vi "main_agv_old.vi"() -> ()   [LabVIEW 2018]
uses:
  Ctrl/SoutWork.ctl
  Ctrl/gps-232.ctl
  Ctrl/gps-databuf.ctl
  Ctrl/obstacle_info.ctl
  Ctrl/waypoint_buf.ctl
  Subvi/global_setting.vi
  <vilib>/imath/engines/lvmath2/RunTimeEngine/Managers/WorkSpace/UID Generator.vi
  <vilib>/imath/engines/lvmath2/RunTimeEngine/RunTimeType/NIMS_RunTimeType_From StrictType (excl LVString).vi
  <instcachedir>/0/NIMS_RunTimeType_From StrictType (excl LVString)_E7E34A65C99947108168652BAD14964D.lvgen/NIMS_RunTimeType_From StrictType (excl LVString)_E7E34A65C99947108168652BAD14964D_000.vi
  <vilib>/imath/engines/lvmath2/RunTimeEngine/LocalVariableDefStatement/MC_LocalVariableDefStatement_Display.vi
  <vilib>/imath/engines/lvmath2/RunTimeEngine/Managers/SymbolTable/Clear UID.vi
  <vilib>/imath/engines/lvmath2/RunTimeEngine/NodeEndStatement/NIMS_NodeEndStatement_Output.vi
  <instcachedir>/0/NIMS_NodeEndStatement_Output_53EC0D466D134D7ABD903AC30B43404B.lvgen/NIMS_NodeEndStatement_Output_53EC0D466D134D7ABD903AC30B43404B_001.vi
  <vilib>/imath/engines/lvmath2/RunTimeEngine/ErrorHandling/NIMS_Finalize Error.vi
  <vilib>/imath/engines/lvmath2/RunTimeEngine/Managers/SymbolTable/NIMS_WorkSpace.lvlib
panel:
  in  "System status":string
  in  "tab":T1(tab)
  in  "starttest":bool
  out "System Feedback":T2={"system state"="normal", "Control Mode"=0, "Battery Voltage (V)"=27.3, "error code High"=0, "error code Low"=0}
  out "AGV_EStop":bool
  out "LiDAR":cluster{sgl[], sgl[]}[](graph)
  out "LiDAR img":T3(plugin-control)
  out "GPS XY Graph":cluster{"X1":dbl, "Y1":dbl}[](graph)
  out "Path":cluster{"pathF4.23":ext[], "pathF4.23":ext[]}[](graph)
  out "Manual":bool
  out "ChoosePath":bool
  out "PathFlag":bool
  out "Obstacle Stop":bool
  out "System Start/Stop":bool
  out "Remote_Stop":bool
  out "Motion Feedback":T4={"Linear Velocity (m/s)"=-0.982, "Angular Velocity (rad/s)"=-0.008} {"Linear Velocity (m/s)" format="%.2f"; "Angular Velocity (rad/s)" format="%.2f"}
  out "Vehicle Motion State":T5
  out "current index":dbl=1036.0 format="%#.1f"
  out "linear velocity":dbl=0.19999999999999996 format="%.2f"
  out "angular velocity":dbl=0.2222269923246912 format="%.2f"
  out "Rotational Vel (rad/s)":dbl min=0.0 max=1.0 step=0.001
  out "Translational Vel (m/s)":dbl min=-1.0 max=1.0 step=0.1
  out "heading=0 alarm":bool
  in  "obstacle limit range":T6={"RL front-x"=1.7, "RL central-x"=1.7, "front-y"=2.0} {"front-y" format="%.1f"}
  out "Image":T3(plugin-control)
  in  "TIM571 IP":string="192.168.0.2"
  in  "TIM571 Mounting Offset":T7={"X_offset[m]"=0.0, "Y_offset[m]"=0.68, "Z_offset[m]"=0.0, "X_Rotation[Deg]"=0.0, "Y_Rotation[Deg]"=180.0, "Z_Rotation[Deg]"=0.0} {"Z_Rotation[Deg]" format="%#.2f"; "Y_Rotation[Deg]" format="%#.2f"; "X_Rotation[Deg]" format="%#.2f"; "Z_offset[m]" format="%#.2f"; "Y_offset[m]" format="%#.2f"; "X_offset[m]" format="%#.2f"}
  in  "vlp-16 range setting":T8={"x range"=20.0, "y range Max"=10.0, "y range Min"=-10.0, "z range"=1.0}
  in  "VLP16 Mounting Offset":T7 {"Z_Rotation[Deg]" format="%#.2f"; "Y_Rotation[Deg]" format="%#.2f"; "X_Rotation[Deg]" format="%#.2f"; "Z_offset[m]" format="%#.2f"; "Y_offset[m]" format="%#.2f"; "X_offset[m]" format="%#.2f"}
  out "LiDAR U8":u8[](array[numeric])
  out "232 buf n":u32(graph)
  out "Heading":dbl=98.684623718
  in  "baud rate gps":u32=115200
  in  "vehicle status":T9
  in  "AGV_Port":refnum<visa-resource-name>="COM5"
  out "Robot Status":T9={"X (m)"=153.55383758084335, "Y (m)"=122.1653462474019, "Z (m)"=9.9059, "Roll (degree)"=-0.425709275, "Pitch (degree)"=-0.898393069, "Heading (degree)"=-8.684623717999997, "Linear velocity (m/s)"=-0.982, "Angular velocity (rad/s)"=-0.008} {"X (m)" format="%.2f"; "Y (m)" format="%#.2f"; "Z (m)" format="%#.2f"; "Roll (degree)" format="%_2g"; "Pitch (degree)" format="%.2f"; "Heading (degree)" format="%.2f"; "Linear velocity (m/s)" format="%.2f"; "Angular velocity (rad/s)" format="%.2f"}
  in  "Remote PC IP":string="223.171.61.153"
  out "Resources":string[][](table)
  out "waypoint graph":T10(graph)
  in  "pathF4.23":ext[][](array[numeric])=array2x4344[8688 elements]
  in  "P2F":ext[][](array[numeric])=array2x2176[4352 elements]
  in  "P1F":ext[][](array[numeric])=array2x2168[4336 elements]
  out "index Y":ext
  out "index X":ext
  out "GNSS Error":errorcluster
  out "IndexPath":ext[][](array[numeric])
  out "Frames/Sec 3":dbl=50.026287540850646 format="%#_2g"
  out "System Feedback code":u8[](array[numeric])=[0, 0, 1, 17, 0, 0]
  out "GPS Data":T11={"Latitude"={"Valid?"=TRUE, "Latitude (Deg)"=37.37123095061}, "Longitude"={"Valid?"=TRUE, "Longitude (Deg)"=126.72256864175}, "Height"={"Valid?"=TRUE, "Height (m)"=9.9059}, "Undulation"={"Valid?"=TRUE, "Undulation(m)"=22.3}, "North Vel"={"Valid?"=TRUE, "North Vel (m/s)"=-0.0013}, "East Vel"={"Valid?"=TRUE, "East Vel (m/s)"=-0.002}, "Up Vel"={"Valid?"=TRUE, "Up Vel (m/s)"=0.0004}, "Roll"={"Valid?"=TRUE, "Roll (degrees)"=-0.425709275}, "Pitch"={"Valid?"=TRUE, "Pitch (degrees)"=-0.898393069}, "Azimuth"={"Valid?"=TRUE, "Azimuth (degrees)"=98.594488749}, "Lat deviation"={"Valid?"=TRUE, "Lat deviation (m)"=0.4755}, "Long deviation"={"Valid?"=TRUE, "Long deviation (m)"=0.4754}, "Height deviation"={"Valid?"=TRUE, "Height deviation (m)"=0.9034}, "North vel deviation"={"Valid?"=TRUE, "North vel deviation (m/s)"=0.0181}, "East vel deviation"={"Valid?"=TRUE, "East vel deviation (m/s)"=0.018}, "Up vel deviation"={"Valid?"=TRUE, "Up vel deviation (m/s)"=0.0196}, "Roll deviation"={"Valid?"=TRUE, "Roll deviation (degrees)"=0.0309}, "Pitch deviation"={"Valid?"=TRUE, "Pitch deviation (degrees)"=0.0311}, "Azimuth deviation"={"Valid?"=TRUE, "Azimuth deviation (degrees)"=0.1368}, "Ext sol status"={"Valid?"=TRUE, "Ext sol status"=0.0}}
  in  "stop":bool
  # "GNSS"
  # "Mando Patrol robot"
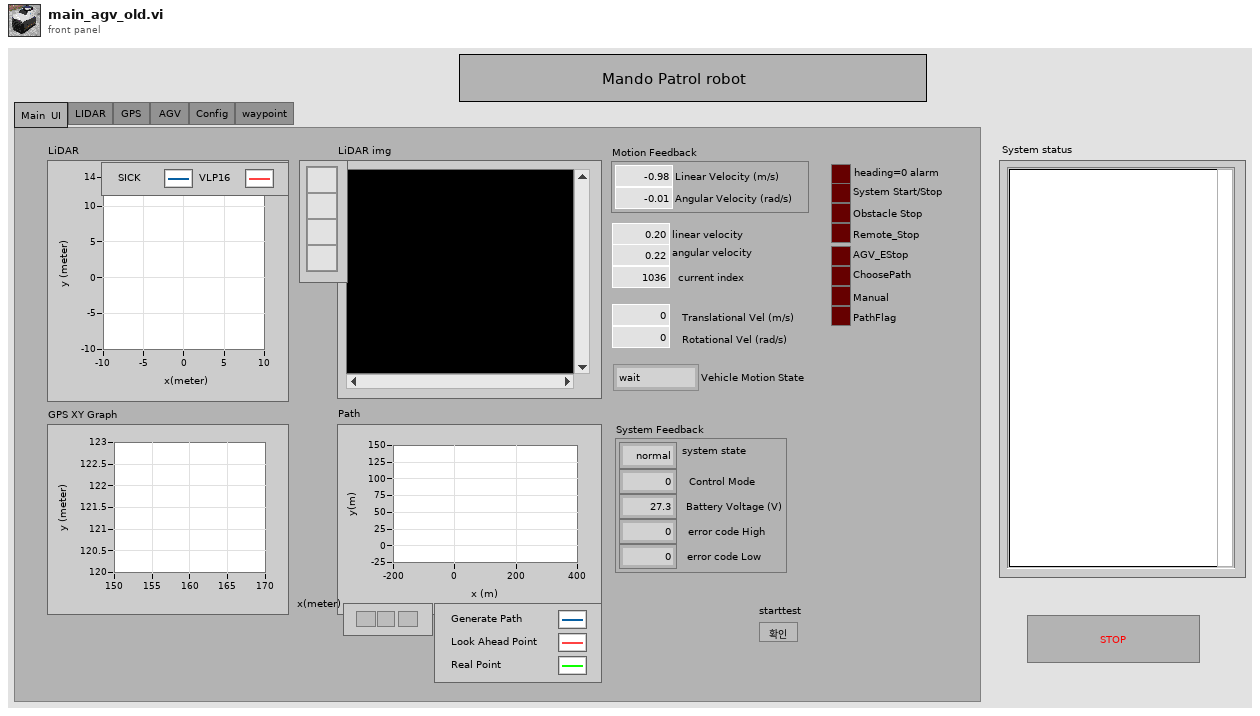
[diagram p1: front panel]
types:
  T1 = enum32{"Main  UI", "LIDAR", "GPS ", "AGV ", "Config", "waypoint"}
  T2 = cluster{"system state":string, "Control Mode":u8, "Battery Voltage (V)":dbl, "error code High":u8, "error code Low":u8}
  T3 = typedef "IMAQ Image.ctl" = refnum<image>
  T4 = cluster{"Linear Velocity (m/s)":dbl, "Angular Velocity (rad/s)":dbl}
  T5 = typedef "SoutWork.ctl" = enum16{"wait", "Move", "ObstacleStop", "EStop", "Goal"}
  T6 = cluster{"RL front-x":dbl, "RL central-x":dbl, "front-y":dbl}
  T7 = cluster{"X_offset[m]":sgl, "Y_offset[m]":sgl, "Z_offset[m]":sgl, "X_Rotation[Deg]":sgl, "Y_Rotation[Deg]":sgl, "Z_Rotation[Deg]":sgl}
  T8 = cluster{"x range":dbl, "y range Max":dbl, "y range Min":dbl, "z range":dbl}
  T9 = cluster{"X (m)":dbl, "Y (m)":dbl, "Z (m)":dbl, "Roll (degree)":dbl, "Pitch (degree)":dbl, "Heading (degree)":dbl, "Linear velocity (m/s)":dbl, "Angular velocity (rad/s)":dbl}
  T10 = cluster{"waypoint out":cluster{"x":dbl, "y":dbl}[]}[]
  T11 = cluster{"Latitude":cluster{"Valid?":bool, "Latitude (Deg)":dbl}, "Longitude":cluster{"Valid?":bool, "Longitude (Deg)":dbl}, "Height":cluster{"Valid?":bool, "Height (m)":dbl}, "Undulation":cluster{"Valid?":bool, "Undulation(m)":dbl}, "North Vel":cluster{"Valid?":bool, "North Vel (m/s)":dbl}, "East Vel":cluster{"Valid?":bool, "East Vel (m/s)":dbl}, "Up Vel":cluster{"Valid?":bool, "Up Vel (m/s)":dbl}, "Roll":cluster{"Valid?":bool, "Roll (degrees)":dbl}, "Pitch":cluster{"Valid?":bool, "Pitch (degrees)":dbl}, "Azimuth":cluster{"Valid?":bool, "Azimuth (degrees)":dbl}, "Lat deviation":cluster{"Valid?":bool, "Lat deviation (m)":dbl}, "Long deviation":cluster{"Valid?":bool, "Long deviation (m)":dbl}, "Height deviation":cluster{"Valid?":bool, "Height deviation (m)":dbl}, "North vel deviation":cluster{"Valid?":bool, "North vel deviation (m/s)":dbl}, "East vel deviation":cluster{"Valid?":bool, "East vel deviation (m/s)":dbl}, "Up vel deviation":cluster{"Valid?":bool, "Up vel deviation (m/s)":dbl}, "Roll deviation":cluster{"Valid?":bool, "Roll deviation (degrees)":dbl}, "Pitch deviation":cluster{"Valid?":bool, "Pitch deviation (degrees)":dbl}, "Azimuth deviation":cluster{"Valid?":bool, "Azimuth deviation (degrees)":dbl}, "Ext sol status":cluster{"Valid?":bool, "Ext sol status":dbl}}
  T12 = typedef "gps-232.ctl" = enum16{"ini", "timing set", "read", "write", "close"}
  T13 = enum16{"write mounting offset", "write range setting", "read"}
  T14 = typedef "obstacle_info.ctl" = enum16{"init", "read", "obstacle status in", "write limit"}
  T15 = typedef "operation.ctl" = enum16{"init", "move", "start pt", "end pt", "start heading adjust", "move heading adjust"}
  T16 = cluster{"VLP16":cluster{"Range setting":cluster{"x range":dbl, "y range Max":dbl, "y range Min":dbl, "z range":dbl}, "Mounting Offset":cluster{"X_offset[m]":sgl, "Y_offset[m]":sgl, "Z_offset[m]":sgl, "X_Rotation[Deg]":sgl, "Y_Rotation[Deg]":sgl, "Z_Rotation[Deg]":sgl}}, "TIM571":cluster{"TIM571 IP":string, "TIM571 Mounting Offset":cluster{"X_offset[m]":sgl, "Y_offset[m]":sgl, "Z_offset[m]":sgl, "X_Rotation[Deg]":sgl, "Y_Rotation[Deg]":sgl, "Z_Rotation[Deg]":sgl}}, "Devices":string[][], "Scout":cluster{"scout port":refnum<visa-resource-name>, "limit_linear-v":dbl, "limit_angular-v":dbl}, "PwrPak7":cluster{"PwrPak7 port":refnum<visa-resource-name>}, "PID":cluster{"PID gains":cluster{"proportional gain (Kc)":dbl, "integral time (Ti, min)":dbl, "derivative time (Td, min)":dbl}, "PID limits":cluster{"output high":dbl, "output low":dbl}, "dt pid":i64}, "Waypoint":cluster{"lookahead pts n":dbl, "lookahead length":dbl}, "obstacle limit range":cluster{"RL front-x":dbl, "RL central-x":dbl, "front-y":dbl}, "System state":cluster{"angle adjust limit":dbl, "State":T15}}
  T17 = cluster{"TIM571 IP":string, "TIM571 Mounting Offset":cluster{"X_offset[m]":sgl, "Y_offset[m]":sgl, "Z_offset[m]":sgl, "X_Rotation[Deg]":sgl, "Y_Rotation[Deg]":sgl, "Z_Rotation[Deg]":sgl}}
  T18 = cluster{"Translational Vel (m/s)":dbl, "Rotational Vel (rad/s)":dbl}
  T19 = cluster{"linear velocity":dbl, "angular velocity":dbl}
  T20 = typedef "gps-databuf.ctl" = enum16{"read", "write"}
  T21 = typedef "waypoint_buf.ctl" = enum16{"clear", "write", "read"}
  T22 = cluster{"rawdata":string, "GPS Data":cluster{"Latitude":cluster{"Valid?":bool, "Latitude (Deg)":dbl}, "Longitude":cluster{"Valid?":bool, "Longitude (Deg)":dbl}, "Height":cluster{"Valid?":bool, "Height (m)":dbl}, "Undulation":cluster{"Valid?":bool, "Undulation(m)":dbl}, "North Vel":cluster{"Valid?":bool, "North Vel (m/s)":dbl}, "East Vel":cluster{"Valid?":bool, "East Vel (m/s)":dbl}, "Up Vel":cluster{"Valid?":bool, "Up Vel (m/s)":dbl}, "Roll":cluster{"Valid?":bool, "Roll (degrees)":dbl}, "Pitch":cluster{"Valid?":bool, "Pitch (degrees)":dbl}, "Azimuth":cluster{"Valid?":bool, "Azimuth (degrees)":dbl}, "Lat deviation":cluster{"Valid?":bool, "Lat deviation (m)":dbl}, "Long deviation":cluster{"Valid?":bool, "Long deviation (m)":dbl}, "Height deviation":cluster{"Valid?":bool, "Height deviation (m)":dbl}, "North vel deviation":cluster{"Valid?":bool, "North vel deviation (m/s)":dbl}, "East vel deviation":cluster{"Valid?":bool, "East vel deviation (m/s)":dbl}, "Up vel deviation":cluster{"Valid?":bool, "Up vel deviation (m/s)":dbl}, "Roll deviation":cluster{"Valid?":bool, "Roll deviation (degrees)":dbl}, "Pitch deviation":cluster{"Valid?":bool, "Pitch deviation (degrees)":dbl}, "Azimuth deviation":cluster{"Valid?":bool, "Azimuth deviation (degrees)":dbl}, "Ext sol status":cluster{"Valid?":bool, "Ext sol status":dbl}}, "Heading":dbl, "utm-1":cluster{"XN":dbl, "YE":dbl}}
  T23 = cluster{"Latitude (Deg)":dbl, "Longitude (Deg)":dbl}
  T24 = cluster{"waypoint out":cluster{"x":dbl, "y":dbl}[]}
  T25 = cluster{"waypoint out":cluster{"Y(E)":dbl, "X(N)":dbl}[]}[]
  T26 = cluster{u8, "index X":ext, "index Y":ext, "System Start/Stop":bool}
  T27 = cluster{"Real Matrix Element":dbl, "Real Matrix Element":dbl}
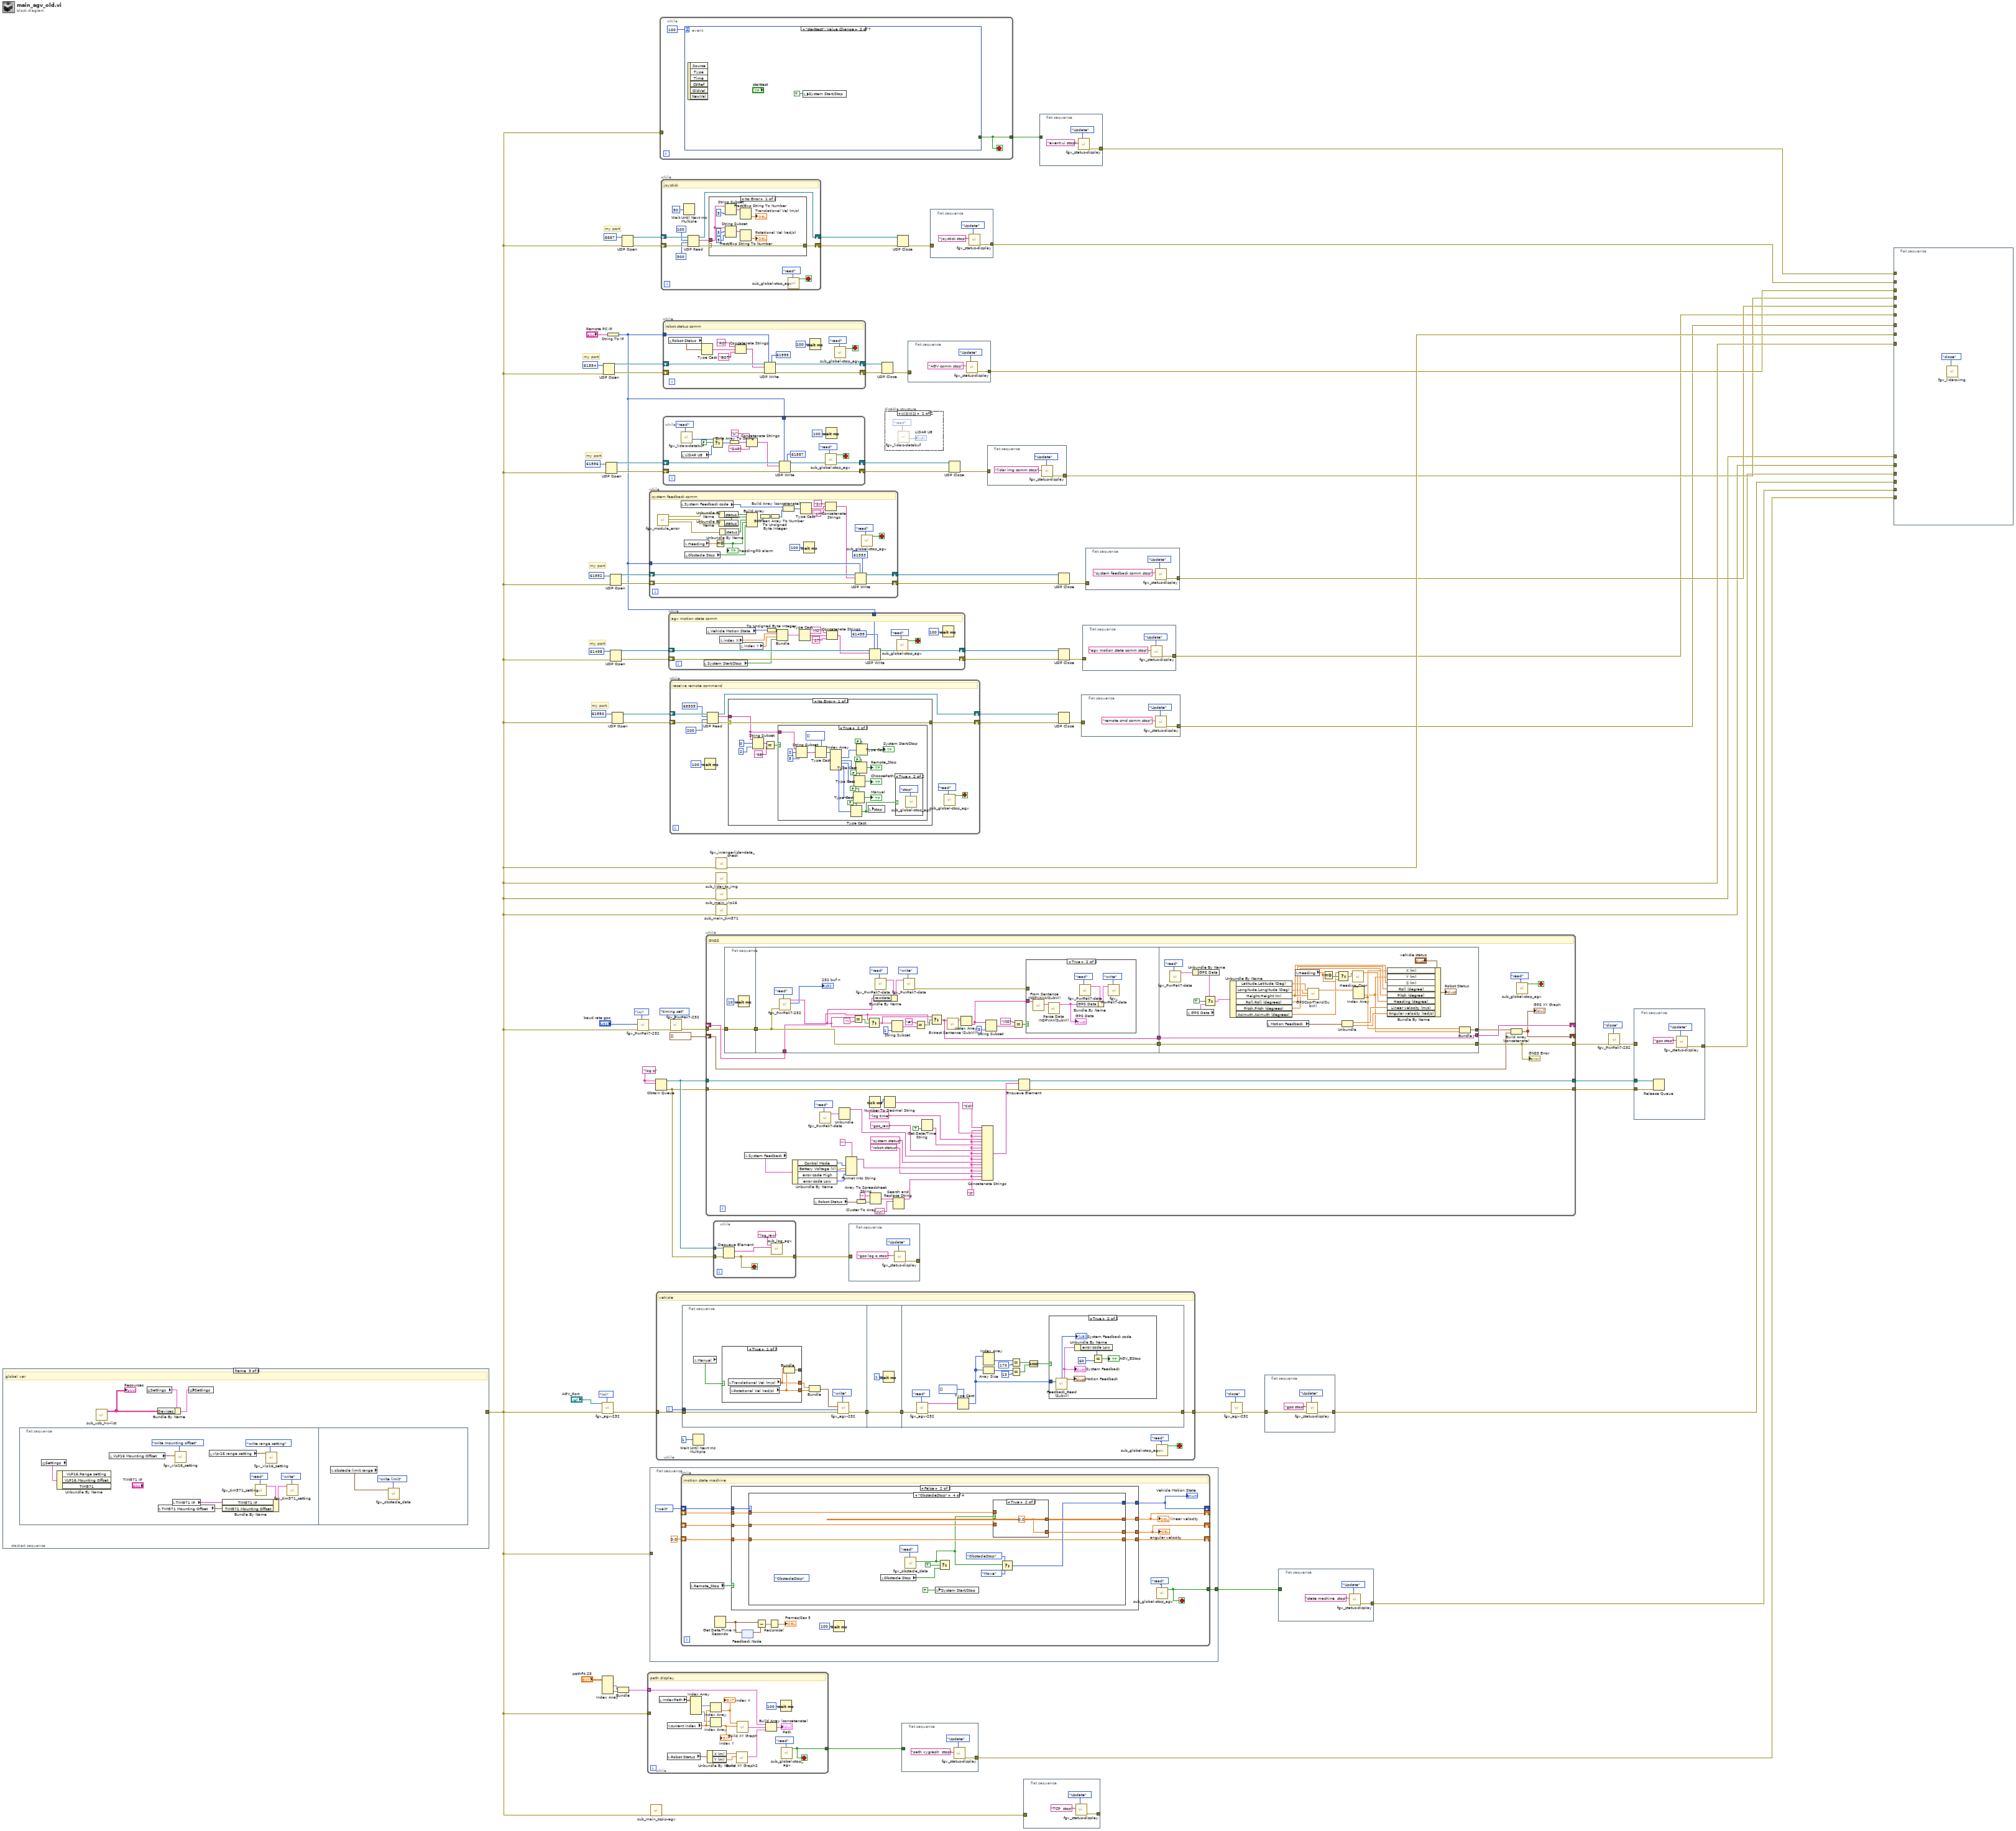
[diagram p0: block diagram]
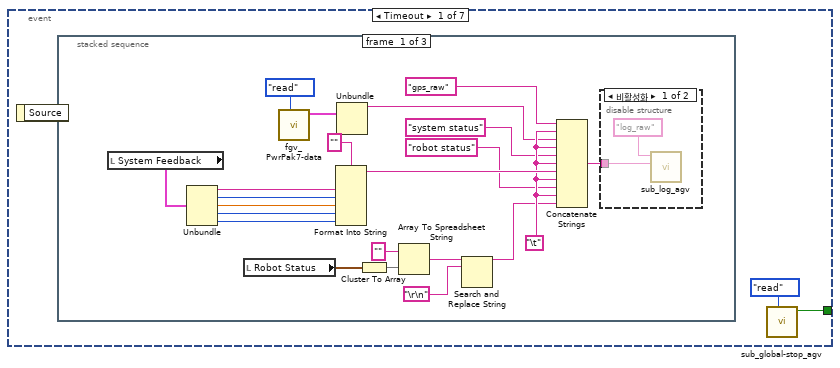
[diagram p3: hidden frame]
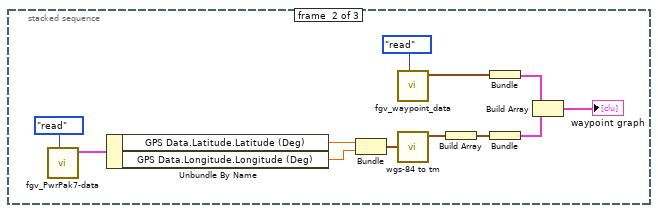
[diagram p5: hidden frame]
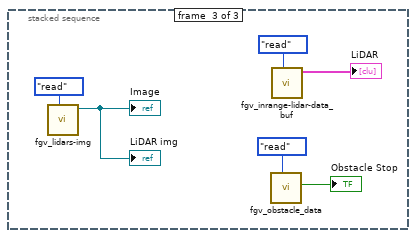
[diagram p6: hidden frame]
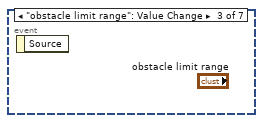
[diagram p7: hidden frame]
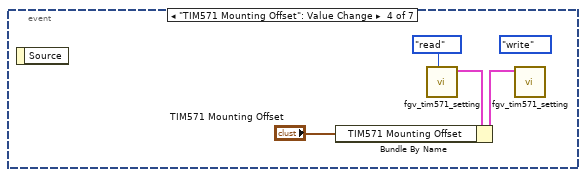
[diagram p8: hidden frame]
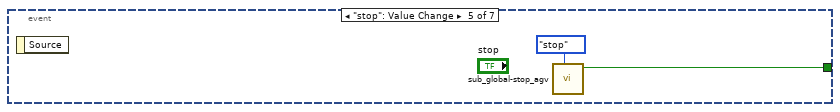
[diagram p9: hidden frame]
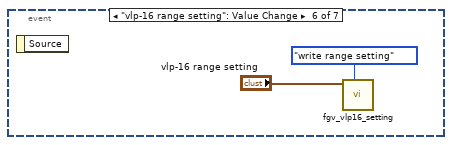
[diagram p10: hidden frame]
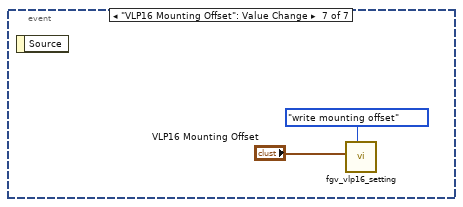
[diagram p11: hidden frame]
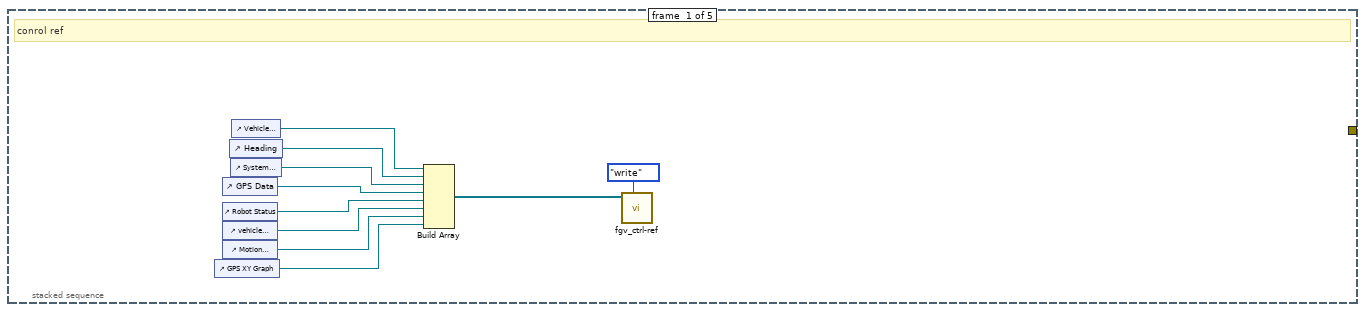
[diagram p12: hidden frame]
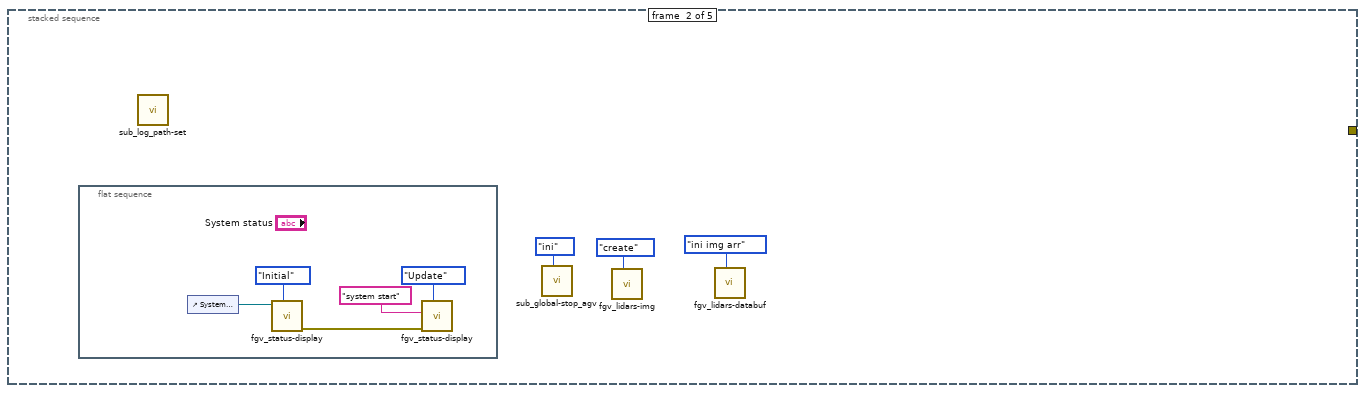
[diagram p13: hidden frame]
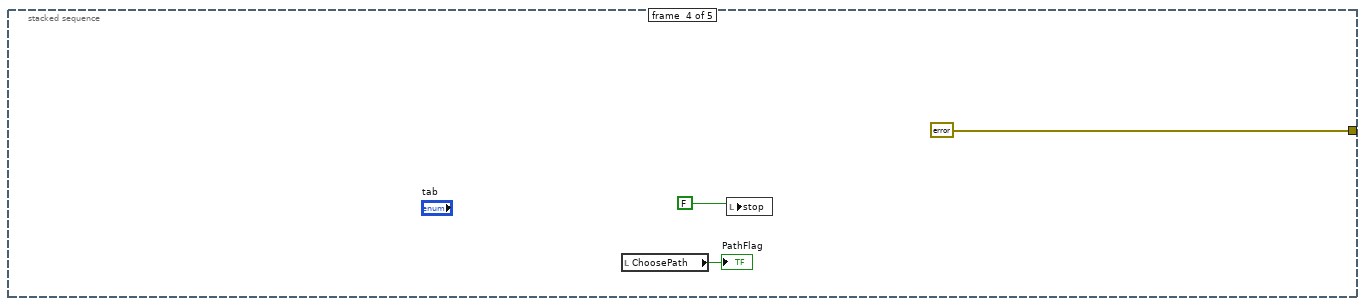
[diagram p14: hidden frame]
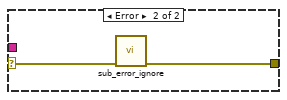
[diagram p16: hidden frame]
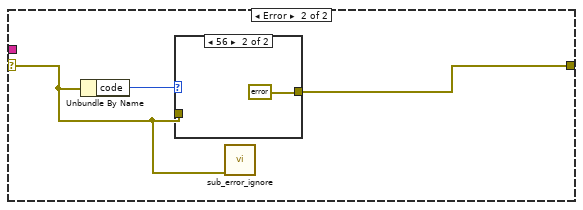
[diagram p19: hidden frame]
diagram:
  w4 = "log q" ("이름(이름없음)")
  # "my port"
  # "my port"
  # "my port"
  # "my port"
  # "my port"
  # "my port"
  n1 = stacked-sequence {
    tunnel: [_ _ _ errorcluster {"status"=FALSE, "code"=0, "source"=""} ("error in (no error)") _] -> w3
    frame #0 {
      # "conrol ref"
      n2 = control-ref of="GPS XY Graph"() -> (w91:refnum<vi>)
      n3 = control-ref of="GPS Data"() -> (w89:refnum<vi>)
      n4 = control-ref of="Robot Status"() -> (w88:refnum<vi>)
      n5 = control-ref of="vehicle status"() -> (w87:refnum<vi>)
      n6 = control-ref of="Motion Feedback"() -> (w90:refnum<vi>)
      n7 = control-ref of="Heading"() -> (w93:refnum<vi>)
      n8 = control-ref of="System status"() -> (w92:refnum<vi>)
      n9 = control-ref of="Vehicle Motion State"() -> (w84:refnum<vi>)
      n10 = Build Array(w84, w93, w92, w89, w88, w87, w90, w91) -> (w86:refnum<vi>[])
      n11 = call "fgv_ctrl-ref.vi"("cmd"=enum16{"write", "read"}."write", "ctrl in"=w86) -> ()  [unwired: 9 in, 1 out]
    }
    frame #1 {
      n12 = flat-sequence {
        frame #0 {
          n13 = control-ref of="System status"() -> (w101:refnum<vi>)
          n14 = call "fgv_status-display.vi"("Mode"=enum16{"Initial", "Update", "Clear"}."Initial", "System Log"=w101) -> ("error out"=w100:errorcluster)  [unwired: 9 in]
          n15 = call "fgv_status-display.vi"("Mode"=enum16{"Initial", "Update", "Clear"}."Update", "error in"=w100, "title"="system start" ("String in 1")) -> ()  [unwired: 8 in, 1 out]
        }
      }
      n16 = call "sub_log_path-set.vi"() -> ()  [unwired: 12 in]
      n17 = call "sub_global-stop_agv.vi"("cmd"=enum16{"ini", "read", "stop"}."ini") -> ()  [unwired: 10 in, 1 out]
      n18 = call "fgv_lidars-img.vi"("cmd"=enum16{"create", "read", "close"}."create") -> ()  [unwired: 10 in, 1 out]
      n19 = call "fgv_lidars-databuf.vi"("cmd"=enum16{"ini img arr", "write", "read"}."ini img arr") -> ()  [unwired: 9 in, 2 out]
    }
    frame #2 {
      # "global var"
      n20 = flat-sequence {
        frame #0 {
          n21 = global read "global_setting.vi" "Settings"() -> (w105:T16)
          n22 = Unbundle By Name(w105) -> ()  [unwired: 3 out]
          n23 = local read "VLP16 Mounting Offset"() -> (w114:T7)
          n24 = local read "TIM571 Mounting Offset"() -> (w109:T7)
          n25 = local read "TIM571 IP"() -> (w111:string)
          n26 = call "fgv_vlp16_setting.vi"("cmd"=T13."write mounting offset", "VLP16 Mounting Offset in"=w114) -> ()  [unwired: 7 in, 3 out]
          n27 = local read "vlp-16 range setting"() -> (w115:T8)
          n28 = call "fgv_tim571_setting.vi"("cmd"=enum16{"write", "read"}."read") -> ("tim571_setting-data_out"=w108:T17)  [unwired: 10 in]
          n29 = Bundle By Name(cluster=w108, "TIM571 IP"=w111, "TIM571 Mounting Offset"=w109) -> (w110:T17)
          n30 = call "fgv_vlp16_setting.vi"("cmd"=T13."write range setting", "vlp-16 range setting in"=w115) -> ()  [unwired: 7 in, 3 out]
          n31 = call "fgv_tim571_setting.vi"("cmd"=enum16{"write", "read"}."write", "tim571_setting-data_in"=w110) -> ()  [unwired: 9 in, 1 out]
        }
        frame #1 {
          n32 = local read "obstacle limit range"() -> (w116:T6)
          n33 = call "fgv_obstacle_data.vi"("cmd"=obstacle_info."write limit", "limit range"=w116) -> ()  [unwired: 7 in, 3 out]
        }
      }
      n34 = call "sub_usb_hw-list.vi"() -> ("Resources"=w104:string[][])  [unwired: 11 in]
      "Resources" <- w104
      n35 = global read "global_setting.vi" "Settings"() -> (w103:T16)
      n36 = Bundle By Name(cluster=w103, "Devices"=w104) -> (w102:T16)
      n37 = global write "global_setting.vi" "Settings"(w102) -> ()
    }
    frame #3 {
      n38 = local read "ChoosePath"() -> (→"PathFlag":bool)
      n39 = local write "stop"(FALSE ("stop")) -> ()
    }
    frame #4 {
    }
  }
  n40 = call "fgv_agv-232.vi"("cmd"=enum16{"ini", "write", "read", "close"}."ini", "error in"=w3, "COM Port"="AGV_Port") -> ("error out"=w78:errorcluster)  [unwired: 6 in, 2 out]
  n41 = Index Array(array="pathF4.23") -> (element #1=w53:ext[], element #2=w52:ext[])  [unwired: 4 in]
  n42 = UDP Open(8:w3, 11:u16 61554 ("port")) -> (port=w74:refnum<k16>, 0:w73:errorcluster)  [unwired: 3 in, 1 out]
  n43 = UDP Open(8:w3, 11:u16 61556 ("port")) -> (port=w80:refnum<k16>, 0:w79:errorcluster)  [unwired: 3 in, 1 out]
  n44 = String To IP(1:"Remote PC IP") -> (0:w49:u32)
  n45 = UDP Open(8:w3, 11:u16 61552 ("port")) -> (port=w68:refnum<k16>, 0:w67:errorcluster)  [unwired: 3 in, 1 out]
  n46 = UDP Open(8:w3, 11:u16 61498 ("port")) -> (port=w58:refnum<k16>, 0:w57:errorcluster)  [unwired: 3 in, 1 out]
  n47 = UDP Open(8:w3, 11:u16 61550 ("port")) -> (port=w63:refnum<k16>, 0:w62:errorcluster)  [unwired: 3 in, 1 out]
  n48 = Bundle("pathF4.23"=w53, "pathF4.23"=w52) -> (w54:cluster{"pathF4.23":ext[], "pathF4.23":ext[]})  [unwired: 1 in]
  n49 = UDP Open(8:w3, 11:u16 6667 ("port")) -> (port=w47:refnum<k16>, 0:w46:errorcluster)  [unwired: 3 in, 1 out]
  n50 = call "fgv_PwrPak7-232.vi"("cmd"=gps-232."ini", "error in"=w3, "baud rate"="baud rate gps") -> ("error out"=w16:errorcluster)  [unwired: 5 in, 3 out]
  n51 = while {
    tunnel: w54 -> [w135]
    tunnel: [w121] -> w31
    tunnel: w3 -> [_]
    stop <- w121 stop-if-true
    # "path display"
    n52 = local read "IndexPath"() -> (w127:ext[][])
    n53 = local read "Robot Status"() -> (w132:T9)
    n54 = local read "current index"() -> (w128:dbl)
    n55 = Index Array(array=w127) -> (element #1=w126:ext[], element #2=w125:ext[])  [unwired: 4 in]
    n56 = Unbundle By Name(w132) -> ("X (m)"=w131:dbl, "Y (m)"=w130:dbl)
    n57 = Index Array(array=w126, index=w128) -> (element=w124:ext)
    "index X" <- w124
    n58 = Index Array(array=w125, index=w128) -> (element=w123:ext)
    "index Y" <- w123
    n59 = call "Build XY Graph2"("Y Input"=w130, "X Input"=w131) -> ("XY Graph"=w129:cluster{"X":dbl[], "Y":dbl[]}[])  [unwired: 8 in, 1 out]
    n60 = call "Build XY Graph"("Y Input"=w123, "X Input"=w124) -> ("XY Graph"=w133:cluster{"X":dbl[], "Y":dbl[]}[])  [unwired: 8 in, 1 out]
    n61 = Build Array (concatenate)(w135, w133, w129) -> (→"Path":cluster{"pathF4.23":ext[], "pathF4.23":ext[]}[])
    n62 = Wait (ms)(milliseconds to wait=u32 100) -> ()  [unwired: 1 out]
    n63 = call "sub_global-stop_agv.vi"("cmd"=enum16{"ini", "read", "stop"}."read") -> ("stop status"=w121:bool)  [unwired: 10 in]
  }
  n64 = while {
    tunnel: w49 -> [w163]
    shift-right: [w160] -> w66
    shift-left: w68 -> [w162]
    shift-right: [w159] -> w65
    shift-left: w67 -> [w161]
    stop <- w140 stop-if-true
    # "system feedback comm"
    n65 = call "fgv_module_error.vi"() -> ("PwrPak7 error out"=w137:errorcluster, "tim571 error out"=w138:errorcluster, "vlp16 error out"=w139:errorcluster)  [unwired: 9 in]
    n66 = local read "System Feedback code"() -> (w153:u8[])
    n67 = local read "Heading"() -> (w145:dbl)
    n68 = local read "Obstacle Stop"() -> (w143:bool)
    n69 = Equal To 0?(x=w145) -> (x = 0?=w144:bool)
    "heading=0 alarm" <- w144
    n70 = Unbundle By Name(w139) -> ("status"=w157:bool)
    n71 = Unbundle By Name(w138) -> ("status"=w156:bool)
    n72 = Unbundle By Name(w137) -> ("status"=w146:bool)
    n73 = Build Array(w157, w156, w146, w144, w143) -> (w155:bool[])
    n74 = Boolean Array To Number(Boolean array=w155) -> (number=w154:u32)
    n75 = To Unsigned Byte Integer(number=w154) -> (unsigned 8bit integer=w152:u8)
    n76 = Build Array (concatenate)(w153, w152) -> (w151:u8[])
    n77 = Type Cast(x=w151) -> (*(type *) &x=w149:string)  [unwired: 1 in]
    n78 = Wait (ms)(milliseconds to wait=u32 100) -> ()  [unwired: 1 out]
    n79 = Concatenate Strings("SY" ("string"), w149, "ST" ("string")) -> (w147:string)
    n80 = UDP Write(address=w163, port or service name=u16 61553, connection ID=w162, data in=w147, 8:w161) -> (error out=w159:errorcluster, 3:w160:refnum<k16>)  [unwired: 1 in]
    n81 = call "sub_global-stop_agv.vi"("cmd"=enum16{"ini", "read", "stop"}."read") -> ("stop status"=w140:bool)  [unwired: 10 in]
  }
  n82 = flat-sequence {
    tunnel: w3 -> [_]
    tunnel: [w164] -> w32
    frame #0 {
      n83 = while {
        shift-right: [w182] -> _
        shift-left: SoutWork."wait" ("열거형") -> [w176]
        shift-right: [w175] -> _
        shift-left: _ -> [w173]
        shift-right: [w174] -> _
        shift-left: _ -> [w172]
        shift-right: [w171] -> _
        shift-left: 0.0 ("current index") -> [w170]
        tunnel: [w167] -> w164
        stop <- w167 stop-if-true
        # "motion state machine"
        n84 = local read "Remote_Stop"() -> (w169:bool)
        n85 = Get Date/Time In Seconds() -> (seconds since 1Jan1904=w180:timestamp)
        n86 = case shown="False" w169 {
          tunnel: [0.0 ("linear velocity") w194] -> w175
          tunnel: [0.0 ("angular velocity") w193] -> w174
          tunnel: w176 -> [_ w192]
          tunnel: [SoutWork."EStop" ("State") w191] -> w182
          tunnel: w173 -> [_ w190]
          tunnel: w172 -> [_ w189]
          tunnel: [w183 w188] -> w171
          tunnel: w170 -> [w183 w187]
          frame True {
          }
          frame False {
            n87 = case shown="\"ObstacleStop\"" w192 {
              tunnel: [w200 w207 0.0 ("linear velocity") w391] -> w194
              tunnel: [w200 w203 0.0 ("linear velocity") w388] -> w193
              tunnel: [w197 SoutWork."ObstacleStop" ("열거형") SoutWork."Goal" ("State") w390] -> w191
              tunnel: w190 -> [_ _ _ w387]
              tunnel: w189 -> [_ _ _ w386]
              tunnel: [w195 w201 w377 w385] -> w188
              tunnel: w187 -> [w195 w206 w377 w385]
              frame "wait", Default {
                w200 = 0.0
                n88 = local read "System Start/Stop"() -> (w196:bool)
                n89 = Select(t=SoutWork."ObstacleStop" ("열거형"), s=w196, f=SoutWork."wait" ("열거형")) -> (s? t:f=w197:T5)
              }
              frame "Move" {
                # "Remote 사용시"
                n90 = local read "PathFlag"() -> (w210:bool)
                n91 = local write "System Start/Stop"(TRUE ("System Start/Stop")) -> ()
                n92 = In Range and Coerce(upper limit=2167.0, x=w206, lower limit=2165.0 ("upper limit")) -> (In Range?=w214:bool)  [unwired: 1 out]
                n93 = Not Or(1:w210, 2:w214) -> (0:w213:bool)
                n94 = case shown="True" w213 {
                  tunnel: ["P1F" "P2F"] -> w209
                  tunnel: w206 -> [w370 w373]
                  tunnel: [w369 w372] -> w205
                  frame True {
                    n95 = formula code="if (i<=750)\nv=0.5;\nelse if (i>750 && i<1550)\nv=0.3;\nelse if (i>=1550 && i<2090)\nv=0.3;\nelse\nv=0.3;\nif (v<0)\nv=0;"("i"=w370) -> ("v"=w369:dbl)
                  }
                  frame False {
                    n96 = formula code="if (i<=30)\nv=0.3;\nelse if (i>30 && i<550)\nv=0.3;\nelse if (i>=550 && i<1420)\nv=0.3;\nelse\nv=0.5;"("i"=w373) -> ("v"=w372:dbl)
                    n97 = local write "PathFlag"(TRUE ("PathFlag")) -> ()
                  }
                }
                "IndexPath" <- w209
                n98 = local read "Robot Status"() -> (w208:T9)
                n99 = call "PurePursuit (SubVI).vi"("target_speed"=w205, "Vehicle Status"=w208, "path"=w209) -> ("linear velocity"=w207:dbl, "angular velocity"=w204:dbl, "current index"=w201:dbl)  [unwired: 14 in]
                "current index" <- w201
                n100 = mathscript code="if (i<300 && i>2100)\n  if (av>0.2)\n   av=0.2\n   else if (av<-0.2)\n   av=-0.2\n   end\n  end\nelse\n  if (av>0.28)\n   av=0.28\n   else if (av<-0.28)\n   av=-0.28\n   end\n  end\nend"("i"=w201, "av"=w204) -> ("av"=w203:dbl)  [unwired: 1 in, 1 out]
              }
              frame "Goal" {
                n101 = local write "System Start/Stop"(FALSE) -> ()
              }
              frame "ObstacleStop" {
                (unwired) SoutWork."ObstacleStop" ("State")
                n102 = local read "Obstacle Stop"() -> (w382:bool)
                n103 = call "fgv_obstacle_data.vi"("cmd"=obstacle_info."read") -> ("obstacle out"=w380:bool)  [unwired: 8 in, 2 out]
                n104 = local write "System Start/Stop"(TRUE ("System Start/Stop")) -> ()
                n105 = Select(t=w380, s=TRUE, f=w382) -> ()  [unwired: 1 out]
                n106 = case shown="True" w380 {
                  tunnel: [w394 w395] -> w391
                  tunnel: [w393 w395] -> w388
                  tunnel: w387 -> [w394 _]
                  tunnel: w386 -> [w393 _]
                  frame False {
                  }
                  frame True {
                    w395 = 0.0 ("linear velocity")
                  }
                }
                n107 = Select(t=SoutWork."ObstacleStop" ("State"), s=w380, f=SoutWork."Move" ("State")) -> (s? t:f=w390:T5)
              }
            }
          }
        }
        "linear velocity" <- w175
        "angular velocity" <- w174
        "Vehicle Motion State" <- w182
        n108 = feedback #1() -> (w179:timestamp)  [unwired: 1 in]
        n109 = feedback-in #1(w180) -> ()
        n110 = Subtract(x=w180, y=w179) -> (x-y=w178:dbl)
        n111 = Reciprocal(x=w178) -> (1/x=→"Frames/Sec 3":dbl)
        n112 = Wait (ms)(milliseconds to wait=u32 100) -> ()  [unwired: 1 out]
        n113 = call "sub_global-stop_agv.vi"("cmd"=enum16{"ini", "read", "stop"}."read") -> ("stop status"=w167:bool)  [unwired: 10 in]
      }
    }
  }
  n114 = call "sub_main_tcpip-agv.vi"("error in"=w3) -> ("error out"=w11:errorcluster)  [unwired: 10 in]
  n115 = Obtain Queue(name (unnamed)=w4, element data type=w4) -> (queue out=w8:refnum<queue>, error out=w7:errorcluster)  [unwired: 3 in, 1 out]
  n116 = while {
    tunnel: w78 -> [w403]
    tunnel: [w401] -> w77
    i -> [w398]
    stop <- w396 stop-if-true
    # "vehicle"
    n117 = flat-sequence {
      tunnel: w403 -> [w408]
      tunnel: w398 -> [w406]
      tunnel: [w407] -> w400
      tunnel: [w418] -> w402
      tunnel: w400 -> [w418]
      tunnel: w402 -> [w420]
      tunnel: [w428] -> w401
      frame #0 {
        n118 = local read "Manual"() -> (w411:bool)
        n119 = case shown="True" w411 {
          tunnel: [w414 w416] -> w410
          tunnel: [w413 w417] -> w409
          tunnel: [w412 w415] -> _
          frame True {
            n120 = local read "Translational Vel (m/s)"() -> (w414:dbl)
            n121 = local read "Rotational Vel (rad/s)"() -> (w413:dbl)
            n122 = Bundle("Translational Vel (m/s)"=w414, "Rotational Vel (rad/s)"=w413) -> (w412:T18)  [unwired: 1 in]
          }
          frame False {
            n123 = local read "angular velocity"() -> (w417:dbl)
            n124 = local read "linear velocity"() -> (w416:dbl)
            n125 = Bundle("linear velocity"=w416, "angular velocity"=w417) -> (w415:T19)  [unwired: 1 in]
          }
        }
        n126 = Bundle("linear velocity"=w410, "angular velocity"=w409) -> (w405:T19)  [unwired: 1 in]
        n127 = call "fgv_agv-232.vi"("cmd"=enum16{"ini", "write", "read", "close"}."write", "error in"=w408, "Frame ID"=w406, "control-val"=w405) -> ("error out"=w407:errorcluster)  [unwired: 5 in, 2 out]
      }
      frame #1 {
        n128 = Wait (ms)(milliseconds to wait=u32 1) -> ()  [unwired: 1 out]
      }
      frame #2 {
        n129 = call "fgv_agv-232.vi"("cmd"=enum16{"ini", "write", "read", "close"}."read", "error in"=w420) -> ("error out"=w428:errorcluster, "read data"=w424:string)  [unwired: 7 in, 1 out]
        n130 = Type Cast(type=i8[] [], x=w424) -> (*(type *) &x=w422:i8[])
        n131 = Index Array(array=w422) -> (element #1=w432:i8)  [unwired: 2 in, 1 out]
        n132 = Array Size(array=w422) -> (size(s)=w430:i32)
        n133 = Equal?(x=w432, y=u8 170) -> (x = y?=w427:bool)
        n134 = Equal?(x=w430, y=13) -> (x = y?=w425:bool)
        n135 = Compound Arithmetic op=AND(w427, w425) -> (w426:bool)
        n136 = case shown="True" w426 {
          tunnel: w422 -> [_ w439]
          frame False {
          }
          frame True {
            n137 = call "Feedback_Read (SubVI).vi"("System State Feedback"=w439) -> ("System Feedback code"=→"System Feedback code":u8[], "System Feedback"=w433:T2, "Motion Feedback"=→"Motion Feedback":T4)  [unwired: 7 in, 5 out]
            "System Feedback" <- w433
            n138 = Unbundle By Name(w433) -> ("error code Low"=w436:u8)
            n139 = Equal?(x=w436, y=u8 60) -> (x = y?=→"AGV_EStop":bool)
          }
        }
      }
    }
    n140 = Wait Until Next ms Multiple(millisecond multiple=i16 1) -> ()  [unwired: 1 out]
    n141 = call "sub_global-stop_agv.vi"("cmd"=enum16{"ini", "read", "stop"}."read") -> ("stop status"=w396:bool)  [unwired: 10 in]
  }
  n142 = while {
    tunnel: w3 -> [_]
    tunnel: [w441] -> w40
    stop <- w441 stop-if-true
    n143 = event shown="[1] \"starttest\": Value Change" {
      selector: _ -> [_ _ _ _ _ _ _]
      dyn-events: _ -> [_ _ _ _ _ _ _]
      timeout: 100 -> [_ _ _ _ _ _ _]
      tunnel: [w442 _ _ _ w491 _ _] -> w441
      event Timeout {
        n144 = event-data() -> ()  [unwired: 1 in, 1 out]
        n145 = stacked-sequence {
          frame #0 {
            w459 = "\t"
            n146 = local read "System Feedback"() -> (w449:T2)
            n147 = Unbundle(w449) -> ("system state"=w448:string, "Control Mode"=w447:u8, "Battery Voltage (V)"=w446:dbl, "error code High"=w445:u8, "error code Low"=w444:u8)
            n148 = local read "Robot Status"() -> (w463:T9)
            n149 = call "fgv_PwrPak7-data.vi"("cmd"=gps-databuf."read") -> ("data cluster out"=w451:T22)  [unwired: 9 in, 1 out]
            n150 = Format Into String(format string="" ("포맷 문자열"), w448, w447, w446, w445, w444) -> (resulting string=w464:string)  [unwired: 2 in, 1 out]
            n151 = Unbundle(w451) -> ("rawdata"=w450:string)  [unwired: 3 out]
            n152 = Cluster To Array(cluster=w463) -> (array=w462:dbl[])
            n153 = Array To Spreadsheet String(array=w462, 3:"" ("포맷 문자열")) -> (spreadsheet string=w455:string)  [unwired: 1 in]
            n154 = Search and Replace String(input string=w455, search string="\r\n") -> (result string=w453:string)  [unwired: 6 in, 3 out]
            n155 = Concatenate Strings("gps_raw" ("포맷 문자열"), w459, w450, w459, "system status" ("포맷 문자열"), w459, w464, w459, "robot status" ("문자열"), w459, w453) -> (w465:string)
            n156 = disable-structure shown="비활성화" {
              disable-tunnel: w465 -> [w467 _]
              frame Disabled {
                n157 = call "sub_log_agv.vi"("desc"=w467, "Title"="log_raw") -> ()  [unwired: 9 in, 1 out]
              }
              frame Enabled {
              }
            }
          }
          frame #1 {
            n158 = call "fgv_PwrPak7-data.vi"("cmd"=gps-databuf."read") -> ("data cluster out"=w471:T22)  [unwired: 9 in, 1 out]
            n159 = Unbundle By Name(w471) -> ("GPS Data.Latitude.Latitude (Deg)"=w472:dbl, "GPS Data.Longitude.Longitude (Deg)"=w473:dbl)
            n160 = Bundle("Latitude (Deg)"=w472, "Longitude (Deg)"=w473) -> (w474:T23)  [unwired: 1 in]
            n161 = call "fgv_waypoint_data.vi"("cmd"=waypoint_buf."read") -> ("waypoint out"=w470:cluster{"x":dbl, "y":dbl}[])  [unwired: 8 in, 2 out]
            n162 = call "wgs-84 to tm.vi"("in_lon-lat"=w474) -> ("TM"=w476:cluster{"Y(E)":dbl, "X(N)":dbl})  [unwired: 10 in]
            n163 = Build Array(w476) -> (w477:cluster{"Y(E)":dbl, "X(N)":dbl}[])
            n164 = Bundle("waypoint out"=w470) -> (w475:T24)  [unwired: 1 in]
            n165 = Bundle(w477) -> (w478:cluster{cluster{"Y(E)":dbl, "X(N)":dbl}[]})  [unwired: 1 in]
            n166 = Build Array(w475, w478) -> (→"waypoint graph":T25)
          }
          frame #2 {
            n167 = call "fgv_lidars-img.vi"("cmd"=enum16{"create", "read", "close"}."read") -> ("New Image"=→"Image" →"LiDAR img":T3)  [unwired: 10 in]
            n168 = call "fgv_obstacle_data.vi"("cmd"=obstacle_info."read") -> ("obstacle out"=→"Obstacle Stop":bool)  [unwired: 8 in, 2 out]
            n169 = call "fgv_inrange-lidar-data_buf.vi"("cmd"=enum16{"read", "write in range lidar"}."read") -> ("in range data out"=→"LiDAR":cluster{sgl[], sgl[]}[])  [unwired: 10 in]
          }
        }
        n170 = call "sub_global-stop_agv.vi"("cmd"=enum16{"ini", "read", "stop"}."read") -> ("stop status"=w442:bool)  [unwired: 10 in]
      }
      event "starttest": Value Change {
        n171 = event-data() -> ()  [unwired: 1 in, 6 out]
        n172 = local write "System Start/Stop"(TRUE ("System Start/Stop")) -> ()
      }
      event "obstacle limit range": Value Change {
        n173 = event-data() -> ()  [unwired: 1 in, 1 out]
      }
      event "TIM571 Mounting Offset": Value Change {
        (unwired) enum16{"write", "read"}."write" ("cmd")
        n174 = event-data() -> ()  [unwired: 1 in, 1 out]
        n175 = call "fgv_tim571_setting.vi"("cmd"=enum16{"write", "read"}."read") -> ("tim571_setting-data_out"=w489:T17)  [unwired: 10 in]
        n176 = Bundle By Name(cluster=w489, "TIM571 Mounting Offset"="TIM571 Mounting Offset") -> (w490:T17)
        n177 = call "fgv_tim571_setting.vi"("tim571_setting-data_in"=w490) -> ()  [unwired: 10 in, 1 out]
      }
      event "stop": Value Change {
        n178 = event-data() -> ()  [unwired: 1 in, 1 out]
        n179 = call "sub_global-stop_agv.vi"("cmd"=enum16{"ini", "read", "stop"}."stop") -> ("stop status"=w491:bool)  [unwired: 10 in]
      }
      event "vlp-16 range setting": Value Change {
        n180 = event-data() -> ()  [unwired: 1 in, 1 out]
        n181 = call "fgv_vlp16_setting.vi"("cmd"=T13."write range setting", "vlp-16 range setting in"="vlp-16 range setting") -> ()  [unwired: 7 in, 3 out]
      }
      event "VLP16 Mounting Offset": Value Change {
        n182 = event-data() -> ()  [unwired: 1 in, 1 out]
        n183 = call "fgv_vlp16_setting.vi"("cmd"=T13."write mounting offset", "VLP16 Mounting Offset in"="VLP16 Mounting Offset") -> ()  [unwired: 7 in, 3 out]
      }
    }
  }
  n184 = while {
    shift-right: [w505] -> w45
    shift-left: w47 -> [w507]
    shift-right: [w504] -> w44
    shift-left: w46 -> [w506]
    stop <- w497 stop-if-true
    # "joystick"
    n185 = Wait Until Next ms Multiple(millisecond multiple=u32 50) -> ()  [unwired: 1 out]
    n186 = UDP Read(connection ID=w507, max size (548)=100, timeout ms (25000)=500, 8:w506) -> (data out=w499:string, error out=w500:errorcluster, 3:w505:refnum<k16>)  [unwired: 2 out]
    n187 = case shown="No Error" w500 {
      selector: w500 -> [w516 w518]
      tunnel: w499 -> [w508 _]
      tunnel: [w516 w517] -> w504
      frame No Error {
        n188 = String Subset(string=w508, length (rest)=5 ("length (rest)")) -> (substring=w515:string)  [unwired: 1 in]
        n189 = String Subset(string=w508, offset (0)=5, length (rest)=5 ("length (rest)")) -> (substring=w514:string)
        n190 = Fract/Exp String To Number(string=w515) -> (number=→"Translational Vel (m/s)":dbl)  [unwired: 3 in, 1 out]
        n191 = Fract/Exp String To Number(string=w514) -> (number=→"Rotational Vel (rad/s)":dbl)  [unwired: 3 in, 1 out]
      }
      frame Error {
        n192 = call "sub_error_ignore.vi"("error in"=w518) -> ("error out"=w517:errorcluster)  [unwired: 10 in]
      }
    }
    n193 = call "sub_global-stop_agv.vi"("cmd"=enum16{"ini", "read", "stop"}."read") -> ("stop status"=w497:bool)  [unwired: 10 in]
  }
  n194 = while {
    tunnel: w49 -> [w532]
    shift-right: [w529] -> w72
    shift-left: w74 -> [w531]
    shift-right: [w528] -> w71
    shift-left: w73 -> [w530]
    stop <- w519 stop-if-true
    # "robot status comm"
    n195 = local read "Robot Status"() -> (w521:T9)
    n196 = Type Cast(x=w521) -> (*(type *) &x=w523:string)  [unwired: 1 in]
    n197 = Concatenate Strings("RO", w523, "BOT" ("string")) -> (w522:string)
    n198 = UDP Write(address=w532, port or service name=u16 61555, connection ID=w531, data in=w522, 8:w530) -> (error out=w528:errorcluster, 3:w529:refnum<k16>)  [unwired: 1 in]
    n199 = Wait (ms)(milliseconds to wait=u32 100) -> ()  [unwired: 1 out]
    n200 = call "sub_global-stop_agv.vi"("cmd"=enum16{"ini", "read", "stop"}."read") -> ("stop status"=w519:bool)  [unwired: 10 in]
  }
  n201 = while {
    tunnel: w49 -> [w548]
    shift-right: [w550] -> w82
    shift-left: w80 -> [w547]
    shift-right: [w549] -> w81
    shift-left: w79 -> [w546]
    stop <- w539 stop-if-true
    n202 = call "fgv_lidars-databuf.vi"("cmd"=enum16{"ini img arr", "write", "read"}."read") -> ("img-data1d out"=w535:u8[])  [unwired: 9 in, 1 out]
    n203 = local read "LiDAR U8"() -> (w536:u8[])
    n204 = Select(t=w535, s=FALSE, f=w536) -> (s? t:f=w534:u8[])
    n205 = Byte Array To String(unsigned byte array=w534) -> (string=w543:string)
    n206 = Concatenate Strings("LI", w543, "DAR" ("string")) -> (w541:string)
    n207 = UDP Write(address=w548, port or service name=u16 61557, connection ID=w547, data in=w541, 8:w546) -> (error out=w549:errorcluster, 3:w550:refnum<k16>)  [unwired: 1 in]
    n208 = call "sub_global-stop_agv.vi"("cmd"=enum16{"ini", "read", "stop"}."read") -> ("stop status"=w539:bool)  [unwired: 10 in]
    n209 = Wait (ms)(milliseconds to wait=u32 100) -> ()  [unwired: 1 out]
  }
  n210 = while {
    tunnel: w49 -> [w569]
    shift-right: [w566] -> w56
    shift-left: w58 -> [w568]
    shift-right: [w565] -> w55
    shift-left: w57 -> [w567]
    stop <- w551 stop-if-true
    # "agv motion state comm"
    n211 = local read "System Start/Stop"() -> (w554:bool)
    n212 = local read "Vehicle Motion State"() -> (w564:T5)
    n213 = local read "index X"() -> (w556:ext)
    n214 = local read "index Y"() -> (w555:ext)
    n215 = To Unsigned Byte Integer(number=w564) -> (unsigned 8bit integer=w557:u8)
    n216 = Bundle(w557, "index X"=w556, "index Y"=w555, "System Start/Stop"=w554) -> (w553:T26)  [unwired: 1 in]
    n217 = Type Cast(x=w553) -> (*(type *) &x=w562:string)  [unwired: 1 in]
    n218 = Concatenate Strings("MO" ("string"), w562, "ST" ("string")) -> (w560:string)
    n219 = UDP Write(address=w569, port or service name=u16 61499, connection ID=w568, data in=w560, 8:w567) -> (error out=w565:errorcluster, 3:w566:refnum<k16>)  [unwired: 1 in]
    n220 = call "sub_global-stop_agv.vi"("cmd"=enum16{"ini", "read", "stop"}."read") -> ("stop status"=w551:bool)  [unwired: 10 in]
    n221 = Wait (ms)(milliseconds to wait=u32 100) -> ()  [unwired: 1 out]
  }
  n222 = while {
    shift-right: [w572] -> w61
    shift-left: w63 -> [w580]
    shift-right: [w578] -> w60
    shift-left: w62 -> [w579]
    stop <- w570 stop-if-true
    # "receive remote command"
    n223 = Wait (ms)(milliseconds to wait=u32 100) -> ()  [unwired: 1 out]
    n224 = UDP Read(connection ID=w580, max size (548)=65535, timeout ms (25000)=200, 8:w579) -> (data out=w575:string, error out=w576:errorcluster, 3:w572:refnum<k16>)  [unwired: 2 out]
    n225 = case shown="No Error" w576 {
      selector: w576 -> [w587 w610]
      tunnel: w575 -> [w581 _]
      tunnel: [w587 w611] -> w578
      frame No Error {
        n226 = String Subset(string=w581, offset (0)=0, length (rest)=2 ("length (rest)")) -> (substring=w584:string)
        n227 = Equal?(x=w584, y="RE") -> (x = y?=w582:bool)
        n228 = case shown="True" w582 {
          tunnel: w581 -> [_ w608]
          frame False {
          }
          frame True {
            n229 = String Subset(string=w608, offset (0)=2, length (rest)=5 ("length (rest)")) -> (substring=w605:string)
            n230 = Type Cast(type=u8[] [] ("Remote Command"), x=w605) -> (*(type *) &x=w603:u8[])
            n231 = Index Array(array=w603) -> (element #1=w602:u8, element #2=w598:u8, element #3=w595:u8, element #4=w592:u8, element #5=w590:u8)  [unwired: 5 in]
            n232 = Type Cast(type=FALSE, x=w590) -> (*(type *) &x=w588:bool)
            n233 = Type Cast(type=FALSE, x=w592) -> (*(type *) &x=→"Manual":bool)
            n234 = Type Cast(type=FALSE, x=w595) -> (*(type *) &x=→"ChoosePath":bool)
            n235 = Type Cast(type=FALSE, x=w598) -> (*(type *) &x=→"Remote_Stop":bool)
            n236 = Type Cast(type=FALSE, x=w602) -> (*(type *) &x=→"System Start/Stop":bool)
            n237 = local write "stop"(w588) -> ()
            n238 = case shown="True" w588 {
              frame False {
              }
              frame True {
                n239 = call "sub_global-stop_agv.vi"("cmd"=enum16{"ini", "read", "stop"}."stop") -> ()  [unwired: 10 in, 1 out]
              }
            }
          }
        }
      }
      frame Error {
        n240 = Unbundle By Name(w610) -> ("code"=w612:i32)
        n241 = case shown="56" w612 {
          tunnel: w610 -> [w613 _]
          tunnel: [w613 errorcluster {"status"=FALSE, "code"=0, "source"=""} ("error IO")] -> w611
          frame 0, Default {
          }
          frame 56 {
          }
        }
        n242 = call "sub_error_ignore.vi"("error in"=w610) -> ()  [unwired: 10 in, 1 out]
      }
    }
    n243 = call "sub_global-stop_agv.vi"("cmd"=enum16{"ini", "read", "stop"}."read") -> ("stop status"=w570:bool)  [unwired: 10 in]
  }
  n244 = call "fgv_PwrPak7-232.vi"("cmd"=gps-232."timing set", "error in"=w16) -> ("error out"=w43:errorcluster)  [unwired: 6 in, 3 out]
  n245 = while {
    shift-right: [w650] -> _
    shift-left: cluster{"X1":dbl, "Y1":dbl}[] [] -> [w657]
    shift-right: [w655] -> _
    shift-left: _ -> [w656]
    tunnel: [w654] -> w42
    tunnel: w43 -> [w648]
    tunnel: w8 -> [w645]
    tunnel: w7 -> [w617]
    tunnel: [w628] -> w5
    tunnel: [w616] -> w1
    stop <- w646 stop-if-true
    w621 = "\t"
    # "GNSS"
    n246 = flat-sequence {
      tunnel: [w658] -> w649
      tunnel: w648 -> [w658]
      tunnel: w656 -> [w660]
      tunnel: [w667] -> w653
      tunnel: [w670] -> w652
      tunnel: w649 -> [w667]
      tunnel: [w723] -> w654
      tunnel: [w724] -> w655
      tunnel: w653 -> [w723]
      tunnel: w652 -> [w724]
      tunnel: [w722] -> w651
      frame #0 {
        n247 = Wait (ms)(milliseconds to wait=u32 10) -> ()  [unwired: 1 out]
      }
      frame #1 {
        n248 = call "fgv_PwrPak7-232.vi"("cmd"=gps-232."read", "error in"=w667) -> ("serial read buf"=→"232 buf n":u32, "read data"=w663:string)  [unwired: 6 in, 2 out]
        n249 = Equal?(x=w663, y="") -> (x = y?=w677:bool)
        n250 = Select(t=w660, s=w677, f=w663) -> (s? t:f=w679:string)
        n251 = call "fgv_PwrPak7-data.vi"("cmd"=gps-databuf."read") -> ("data cluster out"=w664:T22)  [unwired: 9 in, 1 out]
        n252 = Bundle By Name(cluster=w664, "rawdata"=w663) -> (w662:T22)
        n253 = String Subset(string=w679, length (rest)=1 ("길이(나머지)")) -> (substring=w682:string)  [unwired: 1 in]
        n254 = call "fgv_PwrPak7-data.vi"("cmd"=gps-databuf."write", "data cluster in"=w662) -> ("error out"=w661:errorcluster)  [unwired: 8 in, 1 out]
        n255 = Equal?(x="#", y=w682) -> (x = y?=w680:bool)
        n256 = Select(t=w679, s=w680, f=w660) -> (s? t:f=w670:string)
        n257 = call "Extract Sentence (SubVI).vi"("raw sentences"=w670) -> ("extract sentences"=w676:string[])  [unwired: 10 in]
        n258 = Index Array(array=w676) -> (element=w672:string)  [unwired: 1 in]
        n259 = String Subset(string=w672, length (rest)=3 ("길이(나머지)")) -> (substring=w674:string)  [unwired: 1 in]
        n260 = Equal?(x="INS", y=w674) -> (x = y?=w671:bool)
        n261 = case shown="True" w671 {
          tunnel: w672 -> [w689 w697]
          tunnel: w661 -> [_ _]
          frame False {
            n262 = call "From Sentence DualHeading(SubVI).vi"("Extract Sentence"=w689) -> ("Parse Data Array"=w690:string[])  [unwired: 9 in, 1 out]
            n263 = call "Parse Data DualHeading(SubVI).vi"("Parse Data Array"=w690) -> ("Heading"=w684:dbl)  [unwired: 10 in]
            "Heading" <- w684
            n264 = call "fgv_PwrPak7-data.vi"("cmd"=gps-databuf."read") -> ("data cluster out"=w687:T22)  [unwired: 9 in, 1 out]
            n265 = Bundle By Name(cluster=w687, "Heading"=w684) -> (w688:T22)
            n266 = call "fgv_PwrPak7-data.vi"("cmd"=gps-databuf."write", "data cluster in"=w688) -> ()  [unwired: 8 in, 2 out]
          }
          frame True {
            n267 = call "From Sentence INSPVAXA(SubVI).vi"("Extract Sentence"=w697) -> ("Parse Data Array"=w696:string[])  [unwired: 9 in, 1 out]
            n268 = call "Parse Data INSPVAX(SubVI).vi"("Parse Data Array"=w696) -> ("output cluster"=w691:T11)  [unwired: 10 in]
            "GPS Data" <- w691
            n269 = call "fgv_PwrPak7-data.vi"("cmd"=gps-databuf."read") -> ("data cluster out"=w694:T22)  [unwired: 9 in, 1 out]
            n270 = Bundle By Name(cluster=w694, "GPS Data"=w691) -> (w695:T22)
            n271 = call "fgv_PwrPak7-data.vi"("cmd"=gps-databuf."write", "data cluster in"=w695) -> ()  [unwired: 8 in, 2 out]
          }
        }
      }
      frame #2 {
        n272 = call "fgv_PwrPak7-data.vi"("cmd"=gps-databuf."read") -> ("data cluster out"=w701:T22)  [unwired: 9 in, 1 out]
        n273 = local read "GPS Data"() -> (w702:T11)
        n274 = Unbundle By Name(w701) -> ("GPS Data"=w700:T11)
        n275 = Select(t=w700, s=TRUE, f=w702) -> (s? t:f=w698:T11)
        n276 = Unbundle By Name(w698) -> ("Latitude.Latitude (Deg)"=w712:dbl, "Longitude.Longitude (Deg)"=w711:dbl, "Height.Height (m)"=w721:dbl, "Roll.Roll (degrees)"=w720:dbl, "Pitch.Pitch (degrees)"=w719:dbl, "Azimuth.Azimuth (degrees)"=w706:dbl)
        n277 = local read "Motion Feedback"() -> (w717:T4)
        n278 = local read "Heading"() -> (w705:dbl)
        n279 = call "GPSCoorTrans(SubVI).vi"("Height"=w721, "Longitude"=w711, "Latitude"=w712) -> ("Output"=w708:dbl[])  [unwired: 8 in]
        n280 = Equal To 0?(x=w705) -> (x = 0?=w707:bool)
        n281 = Select(t=w706, s=w707, f=w705) -> (s? t:f=w704:dbl)
        n282 = Unbundle(w717) -> ("Linear Velocity (m/s)"=w716:dbl, "Angular Velocity (rad/s)"=w715:dbl)
        n283 = call "Heading_Coor.vi"("heading (degrees)"=w704) -> ("Heading Coor"=w718:dbl)  [unwired: 10 in]
        n284 = Index Array(array=w708) -> (element #1=w709:dbl, element #2=w710:dbl)  [unwired: 2 in]
        n285 = Bundle By Name(cluster="vehicle status", "X (m)"=w710, "Y (m)"=w709, "Z (m)"=w721, "Roll (degree)"=w720, "Pitch (degree)"=w719, "Heading (degree)"=w718, "Linear velocity (m/s)"=w716, "Angular velocity (rad/s)"=w715) -> (→"Robot Status":T9)
        n286 = Bundle("Real Matrix Element"=w710, "Real Matrix Element"=w709) -> (w722:T27)  [unwired: 1 in]
      }
    }
    n287 = local read "System Feedback"() -> (w615:T2)
    n288 = Unbundle By Name(w615) -> ("Control Mode"=w644:u8, "Battery Voltage (V)"=w643:dbl, "error code High"=w642:u8, "error code Low"=w641:u8)
    n289 = local read "Robot Status"() -> (w639:T9)
    n290 = call "fgv_PwrPak7-data.vi"("cmd"=gps-databuf."read") -> ("data cluster out"=w619:T22)  [unwired: 9 in, 1 out]
    n291 = Unbundle(w619) -> ("rawdata"=w618:string)  [unwired: 3 out]
    n292 = Format Into String(format string="" ("포맷 문자열"), w644, w643, w642, w641) -> (resulting string=w640:string)  [unwired: 2 in, 1 out]
    n293 = Cluster To Array(cluster=w639) -> (array=w638:dbl[])
    n294 = Tick Count (ms)() -> (millisecond timer value=w624:u32)
    n295 = Array To Spreadsheet String(array=w638, 3:"" ("포맷 문자열")) -> (spreadsheet string=w637:string)  [unwired: 1 in]
    n296 = Number To Decimal String(number=w624) -> (decimal integer string=w622:string)  [unwired: 1 in]
    n297 = Search and Replace String(input string=w637, search string="\r\n") -> (result string=w636:string)  [unwired: 6 in, 3 out]
    n298 = Get Date/Time String(want seconds? (F)=TRUE ("초 보이기? (거짓)")) -> (time string=w626:string)  [unwired: 2 in, 1 out]
    n299 = Concatenate Strings("tick" ("문자열"), w621, w622, w621, "log time" ("포맷 문자열"), w621, w626, w621, "gps_raw" ("포맷 문자열"), w621, w618, w621, "system status" ("포맷 문자열"), w621, w640, w621, "robot status" ("문자열"), w621, w636) -> (w629:string)
    n300 = Enqueue Element(queue=w645, element=w629, error in (no error)=w617) -> (queue out=w628:refnum<queue>, error out=w616:errorcluster)  [unwired: 1 in, 1 out]
    n301 = Build Array (concatenate)(w651, w657) -> (w650:cluster{"X1":dbl, "Y1":dbl}[])
    "GPS XY Graph" <- w650
    n302 = call "sub_global-stop_agv.vi"("cmd"=enum16{"ini", "read", "stop"}."read") -> ("stop status"=w646:bool)  [unwired: 10 in]
    "GNSS Error" <- w654
  }
  n303 = while {
    tunnel: w8 -> [w729]
    tunnel: w7 -> [w728]
    tunnel: [w727] -> w6
    stop <- w727 stop-if-true
    n304 = Dequeue Element(queue=w729, error in (no error)=w728) -> (element=w725:string, error out=w727:errorcluster)  [unwired: 1 in, 2 out]
    n305 = call "sub_log_agv.vi"("desc"=w725, "Title"="log_raw") -> ()  [unwired: 9 in, 1 out]
  }
  n306 = call "fgv_inrange-lidar-data_check.vi"("error in"=w3) -> ("error out"=w30:errorcluster)  [unwired: 10 in]
  n307 = call "sub_lidar_to_img.vi"("error in"=w3) -> ("error out"=w29:errorcluster)  [unwired: 10 in]
  n308 = call "sub_main_vlp16.vi"("error in"=w3) -> ("error out"=w2:errorcluster)  [unwired: 10 in]
  n309 = call "sub_main_tim571.vi"("error in"=w3) -> ("error out"=w21:errorcluster)  [unwired: 10 in]
  n310 = flat-sequence {
    tunnel: [w730] -> _
    tunnel: w6 -> [_]
    frame #0 {
      n311 = call "fgv_status-display.vi"("Mode"=enum16{"Initial", "Update", "Clear"}."Update", "title"="gps log q stop" ("String in 1")) -> ("error out"=w730:errorcluster)  [unwired: 9 in]
    }
  }
  n312 = UDP Close(connection ID=w72, 8:w71) -> (error out=w38:errorcluster)  [unwired: 1 out]
  n313 = disable-structure shown="비활성화" {
    frame Disabled {
      n314 = call "fgv_lidars-databuf.vi"("cmd"=enum16{"ini img arr", "write", "read"}."read") -> ("img-data1d out"=→"LiDAR U8":u8[])  [unwired: 9 in, 1 out]
    }
    frame Enabled {
    }
  }
  n315 = UDP Close(connection ID=w45, 8:w44) -> (error out=w39:errorcluster)  [unwired: 1 out]
  n316 = flat-sequence {
    tunnel: w31 -> [_]
    tunnel: [w735] -> w18
    frame #0 {
      n317 = call "fgv_status-display.vi"("Mode"=enum16{"Initial", "Update", "Clear"}."Update", "title"="path xygraph  stop" ("String in 1")) -> ("error out"=w735:errorcluster)  [unwired: 9 in]
    }
  }
  n318 = flat-sequence {
    tunnel: w38 -> [_]
    tunnel: [w738] -> w26
    frame #0 {
      n319 = call "fgv_status-display.vi"("Mode"=enum16{"Initial", "Update", "Clear"}."Update", "title"="AGV comm stop" ("String in 1")) -> ("error out"=w738:errorcluster)  [unwired: 9 in]
    }
  }
  n320 = flat-sequence {
    tunnel: w39 -> [_]
    tunnel: [w741] -> w27
    frame #0 {
      n321 = call "fgv_status-display.vi"("Mode"=enum16{"Initial", "Update", "Clear"}."Update", "title"="joystick stop" ("String in 1")) -> ("error out"=w741:errorcluster)  [unwired: 9 in]
    }
  }
  n322 = UDP Close(connection ID=w82, 8:w81) -> (error out=w37:errorcluster)  [unwired: 1 out]
  n323 = flat-sequence {
    tunnel: w37 -> [_]
    tunnel: [w744] -> w25
    frame #0 {
      n324 = call "fgv_status-display.vi"("Mode"=enum16{"Initial", "Update", "Clear"}."Update", "title"="lidar img comm stop" ("String in 1")) -> ("error out"=w744:errorcluster)  [unwired: 9 in]
    }
  }
  n325 = flat-sequence {
    tunnel: [w747] -> _
    tunnel: w11 -> [_]
    frame #0 {
      n326 = call "fgv_status-display.vi"("Mode"=enum16{"Initial", "Update", "Clear"}."Update", "title"="TCP  stop" ("String in 1")) -> ("error out"=w747:errorcluster)  [unwired: 9 in]
    }
  }
  n327 = flat-sequence {
    tunnel: w40 -> [_]
    tunnel: [w750] -> w28
    frame #0 {
      n328 = call "fgv_status-display.vi"("Mode"=enum16{"Initial", "Update", "Clear"}."Update", "title"="event ui stop" ("String in 1")) -> ("error out"=w750:errorcluster)  [unwired: 9 in]
    }
  }
  n329 = UDP Close(connection ID=w66, 8:w65) -> (error out=w36:errorcluster)  [unwired: 1 out]
  n330 = UDP Close(connection ID=w56, 8:w55) -> (error out=w35:errorcluster)  [unwired: 1 out]
  n331 = UDP Close(connection ID=w61, 8:w60) -> (error out=w34:errorcluster)  [unwired: 1 out]
  n332 = flat-sequence {
    tunnel: w34 -> [_]
    tunnel: [w753] -> w22
    frame #0 {
      n333 = call "fgv_status-display.vi"("Mode"=enum16{"Initial", "Update", "Clear"}."Update", "title"="remote cmd comm stop" ("String in 1")) -> ("error out"=w753:errorcluster)  [unwired: 9 in]
    }
  }
  n334 = flat-sequence {
    tunnel: w35 -> [_]
    tunnel: [w756] -> w23
    frame #0 {
      n335 = call "fgv_status-display.vi"("Mode"=enum16{"Initial", "Update", "Clear"}."Update", "title"="agv motion state comm stop" ("String in 1")) -> ("error out"=w756:errorcluster)  [unwired: 9 in]
    }
  }
  n336 = flat-sequence {
    tunnel: w36 -> [_]
    tunnel: [w759] -> w24
    frame #0 {
      n337 = call "fgv_status-display.vi"("Mode"=enum16{"Initial", "Update", "Clear"}."Update", "title"="system feedback comm stop" ("String in 1")) -> ("error out"=w759:errorcluster)  [unwired: 9 in]
    }
  }
  n338 = call "fgv_agv-232.vi"("cmd"=enum16{"ini", "write", "read", "close"}."close", "error in"=w77) -> ("error out"=w10:errorcluster)  [unwired: 7 in, 2 out]
  n339 = flat-sequence {
    tunnel: [w763] -> w9
    tunnel: w10 -> [w762]
    frame #0 {
      n340 = call "fgv_status-display.vi"("Mode"=enum16{"Initial", "Update", "Clear"}."Update", "error in"=w762, "title"="gps stop" ("String in 1")) -> ("error out"=w763:errorcluster)  [unwired: 8 in]
    }
  }
  n341 = flat-sequence {
    tunnel: w32 -> [_]
    tunnel: [w766] -> w19
    frame #0 {
      n342 = call "fgv_status-display.vi"("Mode"=enum16{"Initial", "Update", "Clear"}."Update", "title"="state machine  stop" ("String in 1")) -> ("error out"=w766:errorcluster)  [unwired: 9 in]
    }
  }
  n343 = call "fgv_PwrPak7-232.vi"("cmd"=gps-232."close", "error in"=w42) -> ("error out"=w33:errorcluster)  [unwired: 6 in, 3 out]
  n344 = flat-sequence {
    tunnel: w33 -> [_]
    tunnel: [w771] -> w20
    tunnel: w5 -> [w770]
    tunnel: w1 -> [w769]
    frame #0 {
      n345 = Release Queue(queue=w770, error in (no error)=w769) -> ()  [unwired: 1 in, 3 out]
      n346 = call "fgv_status-display.vi"("Mode"=enum16{"Initial", "Update", "Clear"}."Update", "title"="gps stop" ("String in 1")) -> ("error out"=w771:errorcluster)  [unwired: 9 in]
    }
  }
  n347 = flat-sequence {
    tunnel: w2 -> [_]
    tunnel: w30 -> [_]
    tunnel: w29 -> [_]
    tunnel: w28 -> [_]
    tunnel: w27 -> [_]
    tunnel: w26 -> [_]
    tunnel: w25 -> [_]
    tunnel: w24 -> [_]
    tunnel: w23 -> [_]
    tunnel: w22 -> [_]
    tunnel: w21 -> [_]
    tunnel: w20 -> [_]
    tunnel: w9 -> [_]
    tunnel: w19 -> [_]
    tunnel: w18 -> [_]
    frame #0 {
      n348 = call "fgv_lidars-img.vi"("cmd"=enum16{"create", "read", "close"}."close") -> ()  [unwired: 10 in, 1 out]
    }
  }
